vi "Set Defaults.vi"(11 "NewEntityTemplate in":refnum<class "Game.lvclass">) -> (3 "NewEntityTemplate out":refnum<class "Game.lvclass">)   [LabVIEW 2020, in "Test.lvlib" / "Game.lvclass"]
uses:
  Game.lvclass
  Game.lvclass/Game.ctl
  <vilib>/IlluminatedG/IG Conditum Base/Conditum/Columns/String/String.lvclass
  <vilib>/IlluminatedG/IG Conditum Base/Conditum/Columns/Boolean/Boolean.lvclass
  <vilib>/IlluminatedG/IG Conditum Base/Conditum/Columns/Double/Double.lvclass
  <vilib>/IlluminatedG/IG Conditum Base/Conditum/Columns/Integer/Integer.lvclass
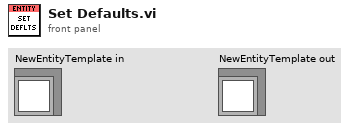
[diagram p1: front panel]
types:
  T1 = typedef "Test.lvlib/Game.lvclass/Columns.ctl" = cluster{"Name":refnum<class "String.lvclass">, "PlayerCount":refnum<class "Integer.lvclass">, "Started":refnum<class "Boolean.lvclass">, "Done":refnum<class "Boolean.lvclass">, "FinalScore":refnum<class "Double.lvclass">}
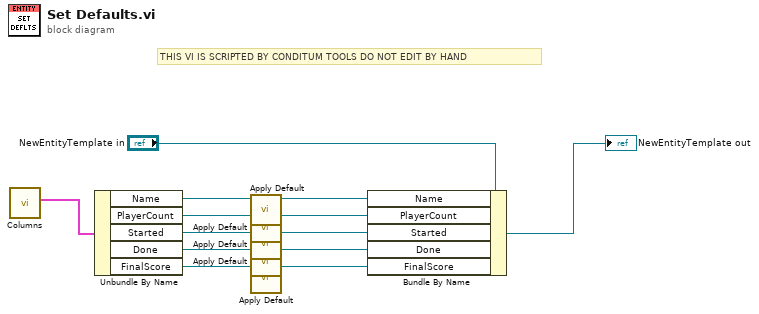
[diagram p0: block diagram]
diagram:
  # "THIS VI IS SCRIPTED BY CONDITUM TOOLS DO NOT EDIT BY HAND"
  n1 = call "Columns.vi"() -> ("Columns"=w13:T1)  [unwired: 11 in]
  n2 = Unbundle By Name(w13) -> ("Name"=w12:refnum<class "String.lvclass">, "PlayerCount"=w8:refnum<class "Integer.lvclass">, "Started"=w7:refnum<class "Boolean.lvclass">, "Done"=w6:refnum<class "Boolean.lvclass">, "FinalScore"=w5:refnum<class "Double.lvclass">)
  n3 = call-dynamic "Apply Default.vi"("String in"=w12) -> ("String out"=w10:refnum<class "String.lvclass">)  [unwired: 10 in]
  n4 = call-dynamic "Apply Default.vi"("Integer in"=w8) -> ("Integer out"=w4:refnum<class "Integer.lvclass">)  [unwired: 10 in]
  n5 = call-dynamic "Apply Default.vi"("Boolean in"=w7) -> ("Boolean out"=w3:refnum<class "Boolean.lvclass">)  [unwired: 10 in]
  n6 = call-dynamic "Apply Default.vi"("Boolean in"=w6) -> ("Boolean out"=w2:refnum<class "Boolean.lvclass">)  [unwired: 10 in]
  n7 = call-dynamic "Apply Default.vi"("Double in"=w5) -> ("Double out"=w1:refnum<class "Double.lvclass">)  [unwired: 10 in]
  n8 = Bundle By Name(cluster="NewEntityTemplate in", "Name"=w10, "PlayerCount"=w4, "Started"=w3, "Done"=w2, "FinalScore"=w1) -> (→"NewEntityTemplate out":refnum<class "Game.lvclass">)
